vi "Create Private Data Control Icon.vi"(11 "Theme Color":u32(colorbox)=255) -> (2 "Icon Out":T1={"image type"=0, "image depth"=24, "image"=array[3072 elements], "mask"=[], "colors"=[], "Rectangle"={"left"=0, "top"=0, "right"=32, "bottom"=32}}, 3 "Icon Image Out":picture)   [LabVIEW 2015, in "QControl Creation.lvclass"]
doc: "<b> </b> <b> </b>\n©2016 Q Software Innovations, LLC (QSI)\nwritten by Quentin Alldredge\nproduced in LabVIEW 2015\n\nsupport@qsoftwareinnovations.com\nwww.qsoftwareinnovations.com\n\nAll rights reserved.\n\nRedistribution and use in source and binary forms, with or without modification, are permitted provided that the following conditions are met:\n\n * Redistributions of source code must retain the above copyright notice, this list of conditions and the following disclaimer.\n * Redistributions in binary form must reproduce the above copyright notice, this list of conditions and the following disclaimer in the documentation and/or other materials provided with the distribution.\n * Neither the name of Q Software Innovations, LLC. nor the names of its contributors may be used to endorse or promote products derived from this software without specific prior written permission.\n\nTHIS SOFTWARE IS PROVIDED BY THE COPYRIGHT HOLDERS AND CONTRIBUTORS \"AS IS\" AND ANY EXPRESS OR IMPLIED WARRANTIES, INCLUDING, BUT NOT LIMITED TO, THE IMPLIED WARRANTIES OF MERCHANTABILITY AND FITNESS FOR A PARTICULAR PURPOSE ARE DISCLAIMED. IN NO EVENT SHALL THE COPYRIGHT OWNER OR CONTRIBUTORS BE LIABLE FOR ANY DIRECT, INDIRECT, INCIDENTAL, SPECIAL, EXEMPLARY, OR CONSEQUENTIAL DAMAGES (INCLUDING, BUT NOT LIMITED TO, PROCUREMENT OF SUBSTITUTE GOODS OR SERVICES; LOSS OF USE, DATA, OR PROFITS; OR BUSINESS INTERRUPTION) HOWEVER CAUSED AND ON ANY THEORY OF LIABILITY, WHETHER IN CONTRACT, STRICT LIABILITY, OR TORT (INCLUDING NEGLIGENCE OR OTHERWISE) ARISING IN ANY WAY OUT OF THE USE OF THIS SOFTWARE, EVEN IF ADVISED OF THE POSSIBILITY OF SUCH DAMAGE."
uses:
  QControl Creation.lvclass
  <vilib>/picture/picture.llb/imagedata.ctl
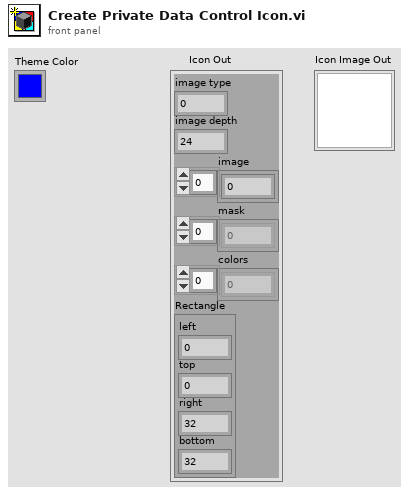
[diagram p1: front panel]
types:
  T1 = typedef "imagedata.ctl" = cluster{"image type":i32, "image depth":i32, "image":u8[], "mask":u8[], "colors":u32[], "Rectangle":cluster{"left":i16, "top":i16, "right":i16, "bottom":i16}}
  T2 = cluster{"left":i16, "top":i16, "right":i16, "bottom":i16}
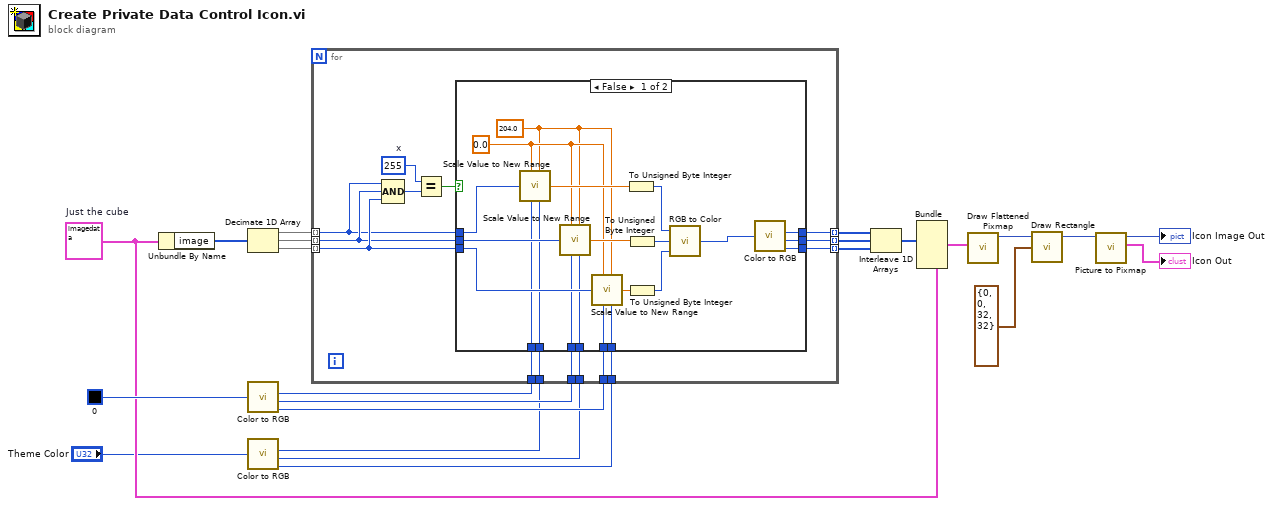
[diagram p0: block diagram]
diagram:
  w7 = T1 {"image type"=0, "image depth"=24, "image"=array[3072 elements], "mask"=[], "colors"=[], "Rectangle"={"left"=0, "top"=0, "right"=32, "bottom"=32}}  # Just the cube
  n1 = Unbundle By Name(w7) -> ("image"=w9:u8[])
  n2 = Decimate 1D Array(w9) -> (w16:u8[], w18:u8[], w17:u8[])
  n3 = call <vilib>:"Color to RGB.vi"("Color"=u32 0) -> ("R"=w12:u8, "G"=w14:u8, "B"=w23:u8)  [unwired: 1 out]
  n4 = call <vilib>:"Color to RGB.vi"("Color"="Theme Color") -> ("R"=w13:u8, "G"=w15:u8, "B"=w22:u8)  [unwired: 1 out]
  n5 = for {
    tunnel: w16 -> [w31] mode=indexing
    tunnel: w18 -> [w32] mode=indexing
    tunnel: w17 -> [w33] mode=indexing
    tunnel: w23 -> [w38]
    tunnel: w22 -> [w37]
    tunnel: [w36] -> w21 mode=indexing
    tunnel: [w35] -> w20 mode=indexing
    tunnel: [w34] -> w19 mode=indexing
    tunnel: w15 -> [w30]
    tunnel: w14 -> [w29]
    tunnel: w13 -> [w28]
    tunnel: w12 -> [w27]
    w25 = u8 255  # x
    n6 = Compound Arithmetic op=AND(w31, w32, w33) -> (w26:u8)
    n7 = Equal?(x=w25, y=w26) -> (x = y?=w24:bool)
    n8 = case shown="False" w24 {
      tunnel: w38 -> [w59 _]
      tunnel: w37 -> [w58 _]
      tunnel: [w57 w62] -> w36
      tunnel: [w56 w61] -> w35
      tunnel: [w55 w60] -> w34
      tunnel: w33 -> [w54 w60]
      tunnel: w32 -> [w53 w61]
      tunnel: w31 -> [w52 w62]
      tunnel: w30 -> [w51 _]
      tunnel: w29 -> [w50 _]
      tunnel: w28 -> [w49 _]
      tunnel: w27 -> [w48 _]
      frame False {
        w43 = 204.0 ("original maximum")
        w44 = 0.0 ("original minimum")
        n9 = call <vilib>:"Scale Value to New Range.vi"("original minimum"=w44, "original value"=w52, "new minimum"=w48, "original maximum"=w43, "new maximum"=w49) -> ("scaled value"=w47:dbl)  [unwired: 4 in]
        n10 = call <vilib>:"Scale Value to New Range.vi"("original minimum"=w44, "original value"=w53, "new minimum"=w50, "original maximum"=w43, "new maximum"=w51) -> ("scaled value"=w46:dbl)  [unwired: 4 in]
        n11 = call <vilib>:"Scale Value to New Range.vi"("original minimum"=w44, "original value"=w54, "new minimum"=w59, "original maximum"=w43, "new maximum"=w58) -> ("scaled value"=w45:dbl)  [unwired: 4 in]
        n12 = To Unsigned Byte Integer(number=w47) -> (unsigned 8bit integer=w42:u8)
        n13 = To Unsigned Byte Integer(number=w46) -> (unsigned 8bit integer=w41:u8)
        n14 = To Unsigned Byte Integer(number=w45) -> (unsigned 8bit integer=w40:u8)
        n15 = call <vilib>:"RGB to Color.vi"("B"=w40, "G"=w41, "R"=w42) -> ("Color"=w39:u32)
        n16 = call <vilib>:"Color to RGB.vi"("Color"=w39) -> ("R"=w57:u8, "G"=w56:u8, "B"=w55:u8)  [unwired: 1 out]
      }
      frame True {
      }
    }
  }
  n17 = Interleave 1D Arrays(w21, w20, w19) -> (w11:u8[])
  n18 = Bundle(cluster=w7, "image"=w11) -> (w8:T1)  [unwired: 5 in]
  n19 = call <vilib>:"Draw Flattened Pixmap.vi"("image data"=w8) -> ("new picture"=w6:picture)  [unwired: 8 in]
  n20 = call <vilib>:"Draw Rectangle.vi"("picture"=w6, "rect"=T2 {"left"=0, "top"=0, "right"=32, "bottom"=32}) -> ("new picture"=w3:picture)  [unwired: 7 in]
  n21 = call <vilib>:"Picture to Pixmap.vi"("picture"=w3) -> ("image data"=→"Icon Out":T1, "new picture"=→"Icon Image Out":picture)  [unwired: 9 in]
